vi "Address Type.vi"(11 "Address In":string) -> (1 "Subnet Bits":i32, 2 "Address":string, 3 "Address Type":T1)   [LabVIEW 2020, in "Vecto.lvlib" / "RemoteDataService.lvclass"]
uses:
  RemoteDataService.lvclass
  RemoteDataService.lvclass/RemoteDataService.ctl
  Address Type.ctl
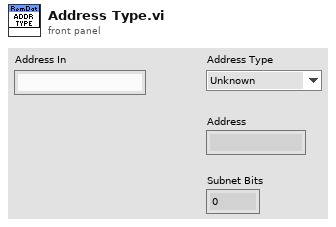
[diagram p1: front panel]
types:
  T1 = typedef "Vecto.lvlib/RemoteDataService.lvclass/Address Type.ctl" = enum16{"Unknown", "Specific", "Subnet", "Any"}
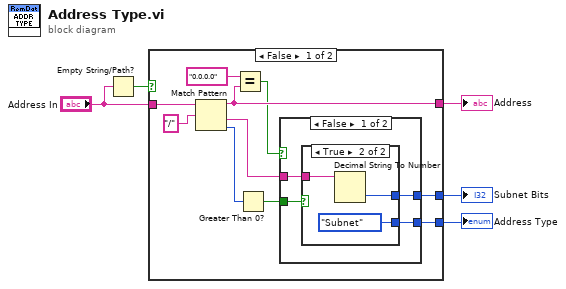
[diagram p0: block diagram]
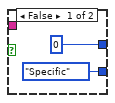
[diagram p2: hidden frame]
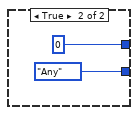
[diagram p3: hidden frame]
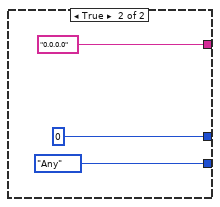
[diagram p4: hidden frame]
diagram:
  n1 = Empty String/Path?(string/path="Address In") -> (empty?=w2:bool)
  n2 = case shown="False" w2 {
    tunnel: "Address In" -> [w13 _]
    tunnel: [w11 0] -> w4
    tunnel: [w10 "0.0.0.0" ("Address In")] -> w3
    tunnel: [w7 Address_Type."Any" ("Address Type")] -> w1
    frame False {
      n3 = Match Pattern(string=w13, regular expression="/") -> (before substring=w10:string, after substring=w12:string, offset past match=w14:i32)  [unwired: 1 in, 1 out]
      n4 = Equal?(x="0.0.0.0", y=w10) -> (x = y?=w8:bool)
      n5 = Greater Than 0?(x=w14) -> (x > 0?=w6:bool)
      n6 = case shown="False" w8 {
        tunnel: w12 -> [w19 _]
        tunnel: [w18 0] -> w11
        tunnel: [w16 Address_Type."Any" ("Address Type")] -> w7
        tunnel: w6 -> [w17 _]
        frame False {
          n7 = case shown="True" w17 {
            tunnel: w19 -> [_ w24]
            tunnel: [0 w23] -> w18
            tunnel: [Address_Type."Specific" ("Address Type") Address_Type."Subnet" ("Address Type")] -> w16
            frame False {
            }
            frame True {
              n8 = Decimal String To Number(string=w24) -> (number=w23:i32)  [unwired: 2 in, 1 out]
            }
          }
        }
        frame True {
        }
      }
    }
    frame True {
    }
  }
  "Address Type" <- w1
  "Address" <- w3
  "Subnet Bits" <- w4
